vi "Reinitialize to defaults.vi"(8 "error in (no error)":errorcluster, 11 "VI Refnum":refnum<vi>) -> (0 "error out":errorcluster)   [LabVIEW 2017, in "Toolbox.lvlib"]
uses:
  Toolbox.lvlib
  Error Handler/Error.lvlib
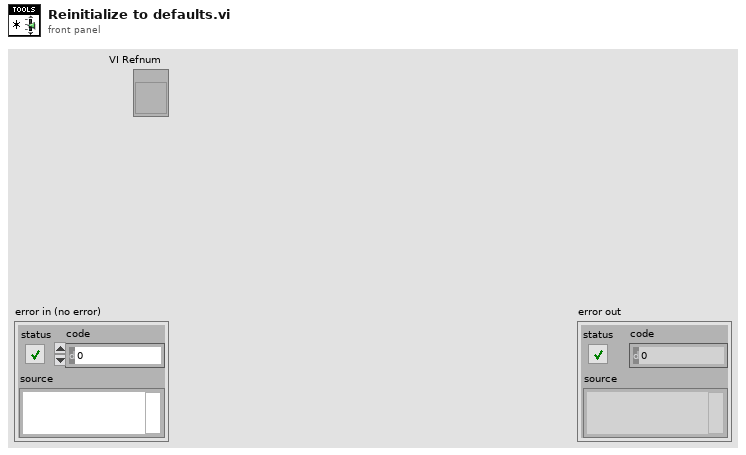
[diagram p1: front panel]
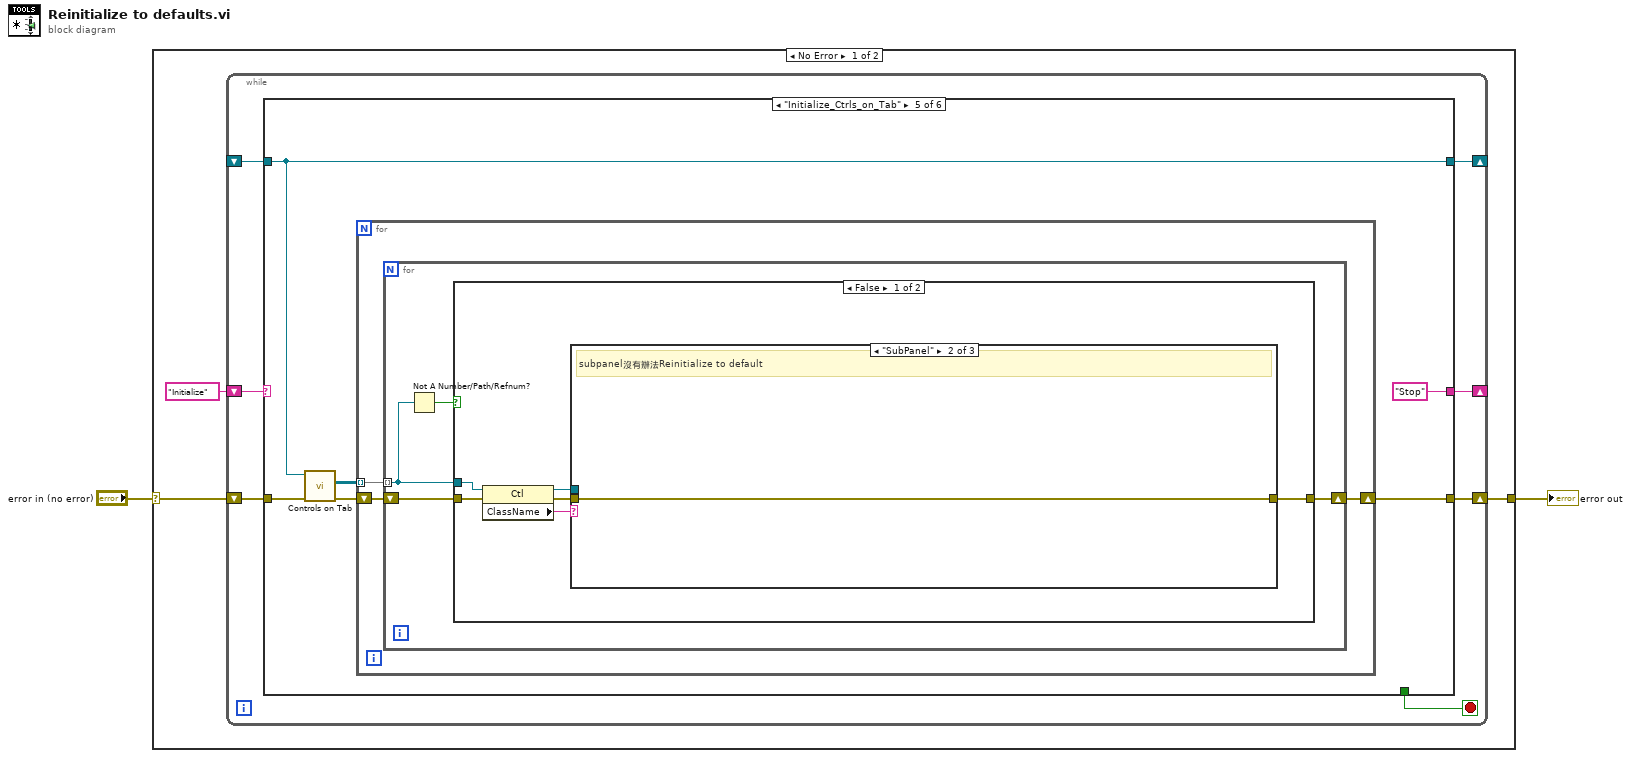
[diagram p0: block diagram]
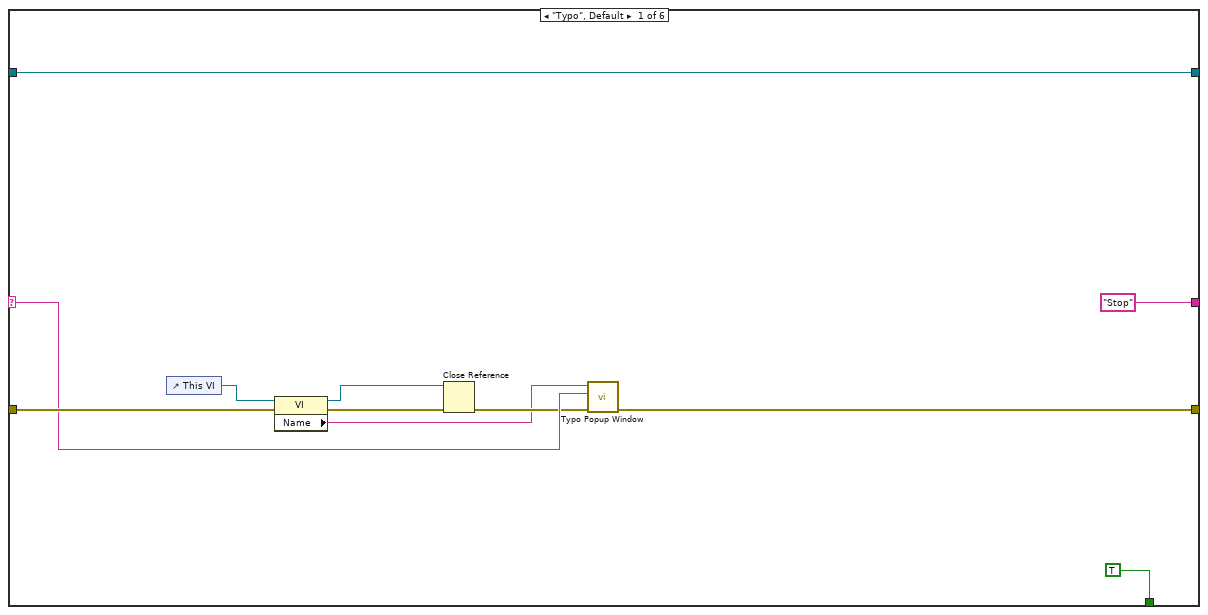
[diagram p2: hidden frame]
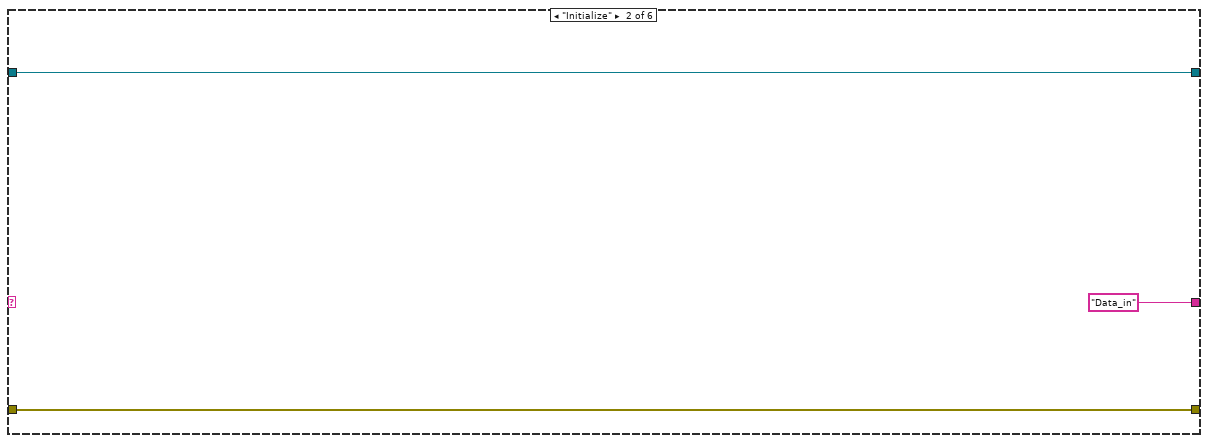
[diagram p3: hidden frame]
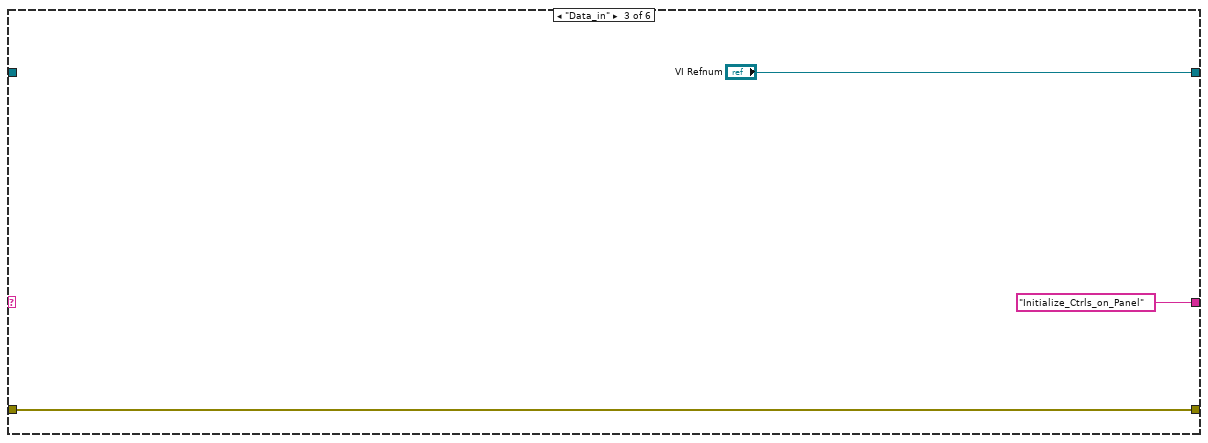
[diagram p4: hidden frame]
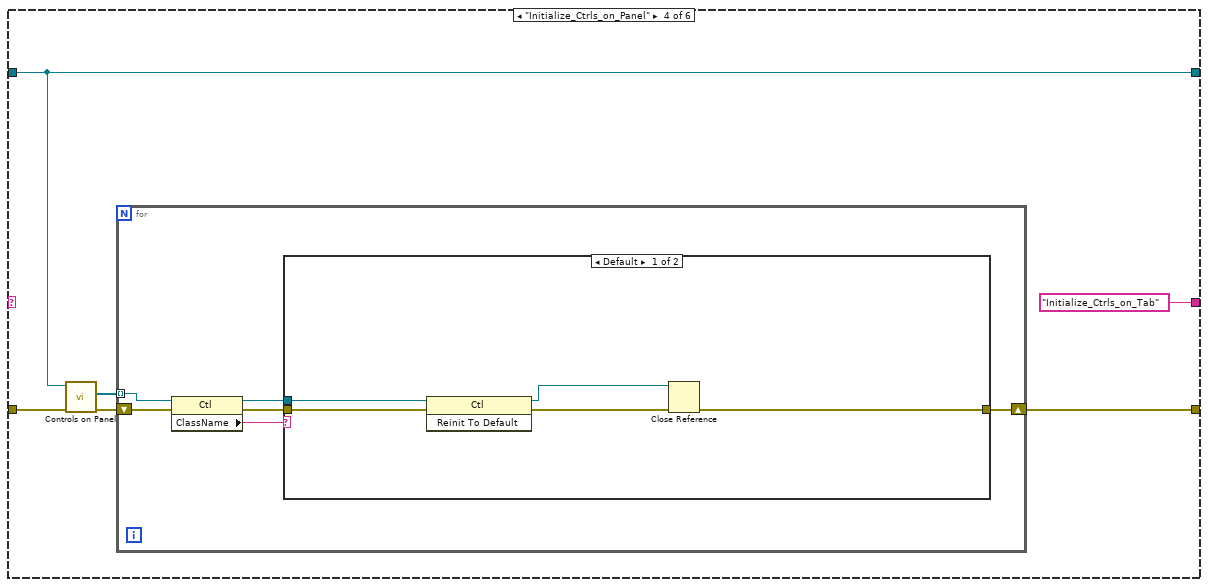
[diagram p5: hidden frame]
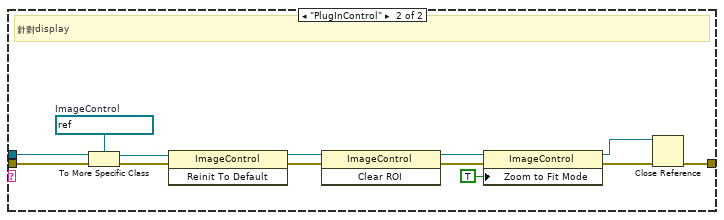
[diagram p6: hidden frame]
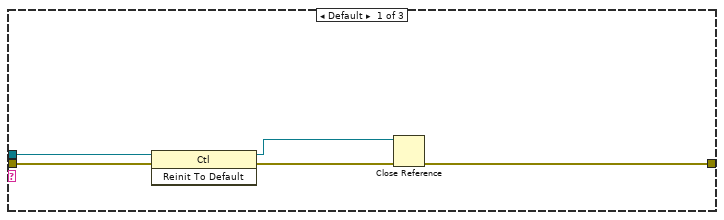
[diagram p7: hidden frame]
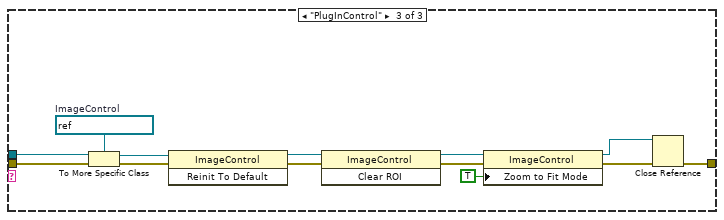
[diagram p8: hidden frame]
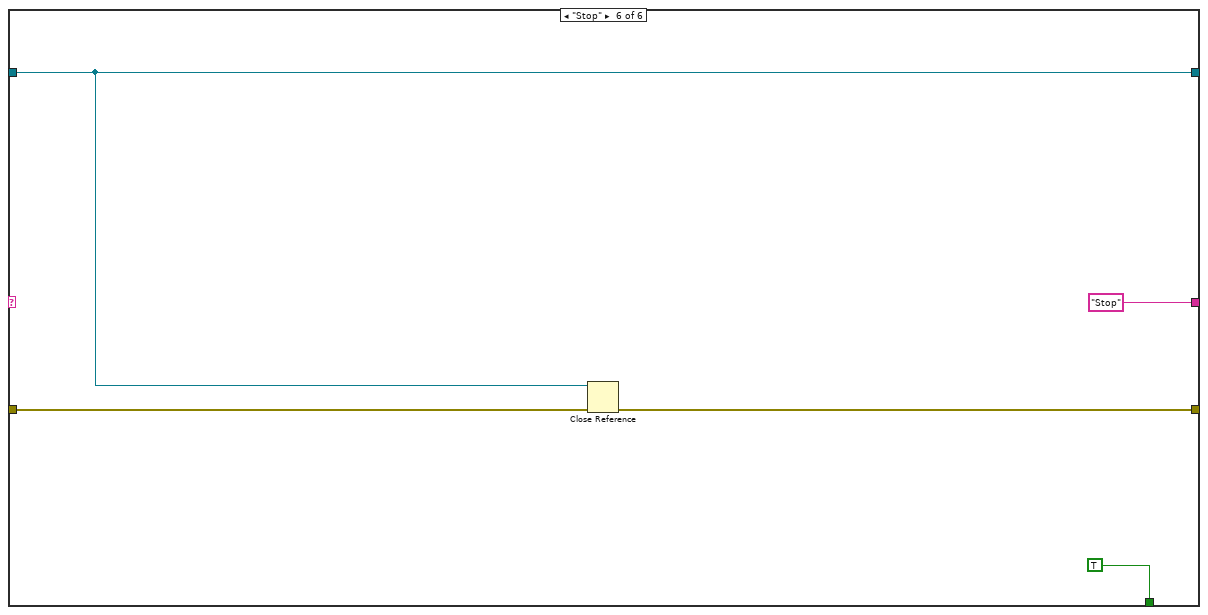
[diagram p10: hidden frame]
diagram:
  n1 = case shown="No Error" "error in (no error)" {
    selector: "error in (no error)" -> [w4 w104]
    tunnel: [w3 w104] -> w1
    frame No Error {
      n2 = while {
        shift-right: [w10] -> w3
        shift-left: w4 -> [w11]
        shift-right: [w9] -> _
        shift-left: "Initialize" -> [w12]
        shift-right: [w7] -> _
        shift-left: _ -> [w6]
        stop <- w8 stop-if-true
        n3 = case shown="\"Initialize_Ctrls_on_Tab\"" w12 {
          selector: w12 -> [w21 _ _ _ _ _]
          tunnel: w11 -> [w23 w26 w29 w35 w65 w103]
          tunnel: [w22 w26 w29 w32 w62 w100] -> w10
          tunnel: ["Stop" "Data_in" "Initialize_Ctrls_on_Panel" "Initialize_Ctrls_on_Tab" "Stop" "Stop"] -> w9
          tunnel: [TRUE _ _ _ _ TRUE] -> w8
          tunnel: [w13 w24 "VI Refnum" w34 w64 w99] -> w7
          tunnel: w6 -> [w13 w24 _ w34 w64 w99]
          frame "Typo", Default {
            n4 = control-ref of="This VI"() -> (w15:refnum<vi>)
            n5 = property class="VI"(reference=w15, error in=w23) -> (reference out=w16:refnum<vi>, error out=w18:errorcluster, "Name"=w14:string)
            n6 = Close Reference(reference=w16, error in (no error)=w18) -> (error out=w17:errorcluster)
            n7 = call "Typo Popup Window.vi"("error in (no error)"=w17, "Typo in"=w21, "VI/Loop name"=w14) -> ("error out"=w22:errorcluster)  [unwired: 8 in]
          }
          frame "Initialize" {
          }
          frame "Data_in" {
          }
          frame "Initialize_Ctrls_on_Panel" {
            n8 = call "Controls on Panel.vi"("error in (no error)"=w35, "VI Refnum in"=w34) -> ("error out"=w33:errorcluster, "ControlOnPanel"=w31:refnum<vi>[])  [unwired: 7 in, 1 out]
            n9 = for {
              shift-right: [w40] -> w32
              shift-left: w33 -> [w41]
              tunnel: w31 -> [w38] mode=indexing
              n10 = property class="Ctl"(reference=w38, error in=w41) -> (reference out=w37:refnum<vi>, error out=w39:errorcluster, "ClassName"=w36:string)
              n11 = case shown="Default" w36 {
                tunnel: w39 -> [w46 w59]
                tunnel: [w45 w49] -> w40
                tunnel: w37 -> [w43 w47]
                frame Default {
                  n12 = invoke class="Ctl" method="Reinit To Default"(reference=w43, error in=w46) -> (reference out=w42:refnum<vi>, error out=w44:errorcluster)  [unwired: 1 in, 1 out]
                  n13 = Close Reference(reference=w42, error in (no error)=w44) -> (error out=w45:errorcluster)
                }
                frame "PlugInControl" {
                  w57 = refnum<vi> refnum  # ImageControl
                  # "針對display"
                  n14 = To More Specific Class(target class=w57, reference=w47, error in=w59) -> (specific class reference=w55:refnum<vi>, error out=w58:errorcluster)
                  n15 = invoke class="ImageControl" method="Reinit To Default"(reference=w55, error in=w58) -> (reference out=w52:refnum<vi>, error out=w56:errorcluster)  [unwired: 1 in, 1 out]
                  n16 = invoke class="ImageControl" method="Clear ROI"(reference=w52, error in=w56) -> (reference out=w51:refnum<vi>, error out=w53:errorcluster)  [unwired: 1 in, 1 out]
                  n17 = property class="ImageControl"(reference=w51, error in=w53, "Zoom to Fit Mode"=TRUE) -> (reference out=w48:refnum<vi>, error out=w54:errorcluster)
                  n18 = Close Reference(reference=w48, error in (no error)=w54) -> (error out=w49:errorcluster)
                }
              }
            }
          }
          frame "Initialize_Ctrls_on_Tab" {
            n19 = call "Controls on Tab.vi"("error in (no error)"=w65, "VI Refnum in"=w64) -> ("error out"=w63:errorcluster, "ControlOnPages"=w61:refnum<vi>[][])  [unwired: 7 in, 1 out]
            n20 = for {
              shift-right: [w67] -> w62
              shift-left: w63 -> [w68]
              tunnel: w61 -> [w66] mode=indexing
              n21 = for {
                shift-right: [w71] -> w67
                shift-left: w68 -> [w72]
                tunnel: w66 -> [w69] mode=indexing
                n22 = Not A Number/Path/Refnum?(number/path/refnum=w69) -> (NaN/Path/Refnum?=w70:bool)
                n23 = case shown="False" w70 {
                  tunnel: w72 -> [w78 w98]
                  tunnel: [w77 w98] -> w71
                  tunnel: w69 -> [w73 _]
                  frame False {
                    n24 = property class="Ctl"(reference=w73, error in=w78) -> (reference out=w75:refnum<vi>, error out=w76:errorcluster, "ClassName"=w74:string)
                    n25 = case shown="\"SubPanel\"" w74 {
                      tunnel: w76 -> [w83 w84 w97]
                      tunnel: [w82 w84 w87] -> w77
                      tunnel: w75 -> [w80 _ w85]
                      frame Default {
                        n26 = invoke class="Ctl" method="Reinit To Default"(reference=w80, error in=w83) -> (reference out=w79:refnum<vi>, error out=w81:errorcluster)  [unwired: 1 in, 1 out]
                        n27 = Close Reference(reference=w79, error in (no error)=w81) -> (error out=w82:errorcluster)
                      }
                      frame "SubPanel" {
                        # "subpanel沒有辦法Reinitialize to default"
                      }
                      frame "PlugInControl" {
                        w95 = refnum<vi> refnum  # ImageControl
                        n28 = To More Specific Class(target class=w95, reference=w85, error in=w97) -> (specific class reference=w93:refnum<vi>, error out=w96:errorcluster)
                        n29 = invoke class="ImageControl" method="Reinit To Default"(reference=w93, error in=w96) -> (reference out=w90:refnum<vi>, error out=w94:errorcluster)  [unwired: 1 in, 1 out]
                        n30 = invoke class="ImageControl" method="Clear ROI"(reference=w90, error in=w94) -> (reference out=w89:refnum<vi>, error out=w91:errorcluster)  [unwired: 1 in, 1 out]
                        n31 = property class="ImageControl"(reference=w89, error in=w91, "Zoom to Fit Mode"=TRUE) -> (reference out=w86:refnum<vi>, error out=w92:errorcluster)
                        n32 = Close Reference(reference=w86, error in (no error)=w92) -> (error out=w87:errorcluster)
                      }
                    }
                  }
                  frame True {
                    # "不同頁簽內control的數量不同\n為了組成array有些reference會變成null"
                  }
                }
              }
            }
          }
          frame "Stop" {
            n33 = Close Reference(reference=w99, error in (no error)=w103) -> (error out=w100:errorcluster)
          }
        }
      }
    }
    frame Error {
    }
  }
  "error out" <- w1
